vi "daqmx watchdog config UI.vi"() -> ()   [LabVIEW 2014, in "DAQmx Watchdog editor node.lvclass"]
doc: "All child modules share this same UI. The UI allows for the configuration of Channels, Parameters, and Error Handling."
uses:
  DAQmx Watchdog editor node.lvclass
  <vilib>/NI/Configuration Framework/Node/NodeRef.ctl
  <vilib>/NI/Configuration Framework/Node/NISE_CEF_Node.lvclass
  <vilib>/NI/AMC/Message Queue.ctl
  <vilib>/NI/AMC/Message.ctl
  <vilib>/NI/Tools/Keyed Array/KeyedArray.ctl
  <vilib>/NI/Configuration Framework/Node/UserEventRef.ctl
  <vilib>/NI/Configuration Framework/Controls/EventCluster.ctl
  <vilib>/NI/DCAF/Tag Editor Core/control module/configuration/error classification setting.ctl
  <vilib>/NI/Tag Bus Module Framework/runtime/error classification.ctl
  <vilib>/NI/Configuration Framework/Node/RefreshUIEvent.ctl
  <vilib>/NI/Configuration Framework/Node/CacheState.ctl
  <vilib>/NI/Configuration Framework/Node/StopEvent.ctl
  <vilib>/NI/Configuration Framework/Node/NodeChangeEvent.ctl
  <vilib>/NI/DCAF/Tag Editor Core/Table API/Available Tag Menu/channel action event.ctl
  <vilib>/NI/DCAF/Tag Editor Core/Table API/Available Tag Menu/dialog output action.ctl
  <vilib>/NI/Tag Bus Module Framework/channel/TBM channel.lvclass
  <vilib>/NI/Tag Bus/tag/tag descriptor.lvclass
  <vilib>/NI/DCAF/Tag Editor Core/Table API/Table Manager/Call Back Ref Type Def.ctl
  <vilib>/NI/DCAF/Tag Editor Core/Configuration Editor/Classes/Engine Parent/Engine Parent Editor Node.lvclass
  <vilib>/NI/DCAF/Tag Editor Core/Configuration Editor/Classes/Module editor node/module editor node.lvclass
  <vilib>/NI/DCAF/Tag Editor Core/Table API/Table Manager/references.ctl
  <vilib>/NI/DCAF/Tag Editor Core/Table API/Table Manager/Menu Definition.ctl
  <vilib>/NI/DCAF/Tag Editor Core/Table API/Table Manager/Menu Options.ctl
  <vilib>/NI/DCAF/Tag Editor Core/control module/configuration/control module configuration.lvclass
  <vilib>/NI/DCAF/Tag Editor Core/Table API/Table Manager/Table Events.ctl
  <vilib>/NI/DCAF/Tag Editor Core/Table API/Table Manager/Menu Select.ctl
  <vilib>/NI/DCAF/Tag Editor Core/control module/editor node/control module editor.lvclass
  <vilib>/NI/DCAF/Tag Editor Core/control module/configuration/control module configuration.lvclass/control module configuration.ctl
  <vilib>/NI/Configuration Framework/serializable configuration/NISE_CEF_serializable configuration.lvclass/NISE_CEF_serializable configuration.ctl
  <vilib>/NI/Tag Bus Module Framework/channel/channel classification.ctl
  module/configuration/DAQmx Watchdog configuration.lvclass
  <vilib>/NI/DCAF/Tag Editor Core/control module/configuration/Write error classifications.vi
  <vilib>/NI/DCAF/Tag Editor Core/Configuration Editor/Classes/Module editor node/Read Module Configuration.vi
  <vilib>/NI/DCAF/Tag Editor Core/control module/editor node/read fixed channel configuration.vi
  <vilib>/Utility/LVClass/Get LV Class Name.vi
  <vilib>/NI/Configuration Framework/error generator/NISE_error generator.vi
  <vilib>/NI/Tag Bus Module Framework/module configuration/TBM module configuration.lvclass
  <vilib>/NI/Configuration Framework/serializable configuration/NISE_CEF_serializable configuration.lvclass
  <vilib>/NI/DCAF/Tag Editor Core/Table API/Listbox/Multi Column Listbox.lvclass
  <vilib>/NI/Configuration Framework/NISE_CEF_TreeControl.lvlib
  <vilib>/NI/DCAF/Tag Editor Core/Table API/Table Manager.lvlib
  <vilib>/NI/DCAF UI Toolkit/Controls/DCAF UI Elements.lvlib
  <vilib>/NI/Tools/Keyed Array/Tools_KeyedArray.lvlib
  <vilib>/NI/AMC/AMC.lvlib
  <vilib>/NI/DCAF/Tag Editor Core/Table API/Table Manager/Table Manager.lvclass
  <vilib>/NI/Tag Bus Module Framework/runtime/TBM module execution interface.lvclass
panel:
  in  "Enum":i32
  in  "user event out":refnum<user-event>
  in  "Top Level Tab Control":enum32{"Watchdog", "Mapping", "Error Handling"}(tab)
  in  "Trigger on network":bool=TRUE
  in  "Digital States":T1(array[cluster]) caption="Digital Output" {"expiration state" items=["High"=10192, "Low"=10214, "Tristate"=10310, "No Change"=10160]}
  in  "Counter States":T1(array[cluster]) caption="Counter Output" {"expiration state" items=["Low"=10214, "High"=10192, "No Change"=10160]}
  in  "Analog States":T2(array[cluster]) caption="Analog Output" {"output type" items=["Voltage"=10322, "Current"=10134, "No Change"=10160]}
  in  "DAQmx Device Name":tag
  in  "Timeout (s)":dbl=0.01 format="%#_13g"
  in  "Edge":i32(ring)=10280 items=["Rising"=10280, "Falling"=10171]
  in  "Trigger Source":tag
  in  "Trigger Type":i32(ring)=10150 items=["Digital Edge"=10150, "Time"=15996]
  in  "Channels Listbox":i32(listbox)
  in  "mapall":bool
  in  "mapwriters":bool
  in  "error classifications":T3[](array[typedef])
  in  "node change":T5
  in  "stop event":T6
  in  "cache state":T7
  in  "refresh UI":T8
  in  "user event":T9
  in  "main queue":T10
  in  "node ref":T11
  # "Triggering"
  # "Expiration States"
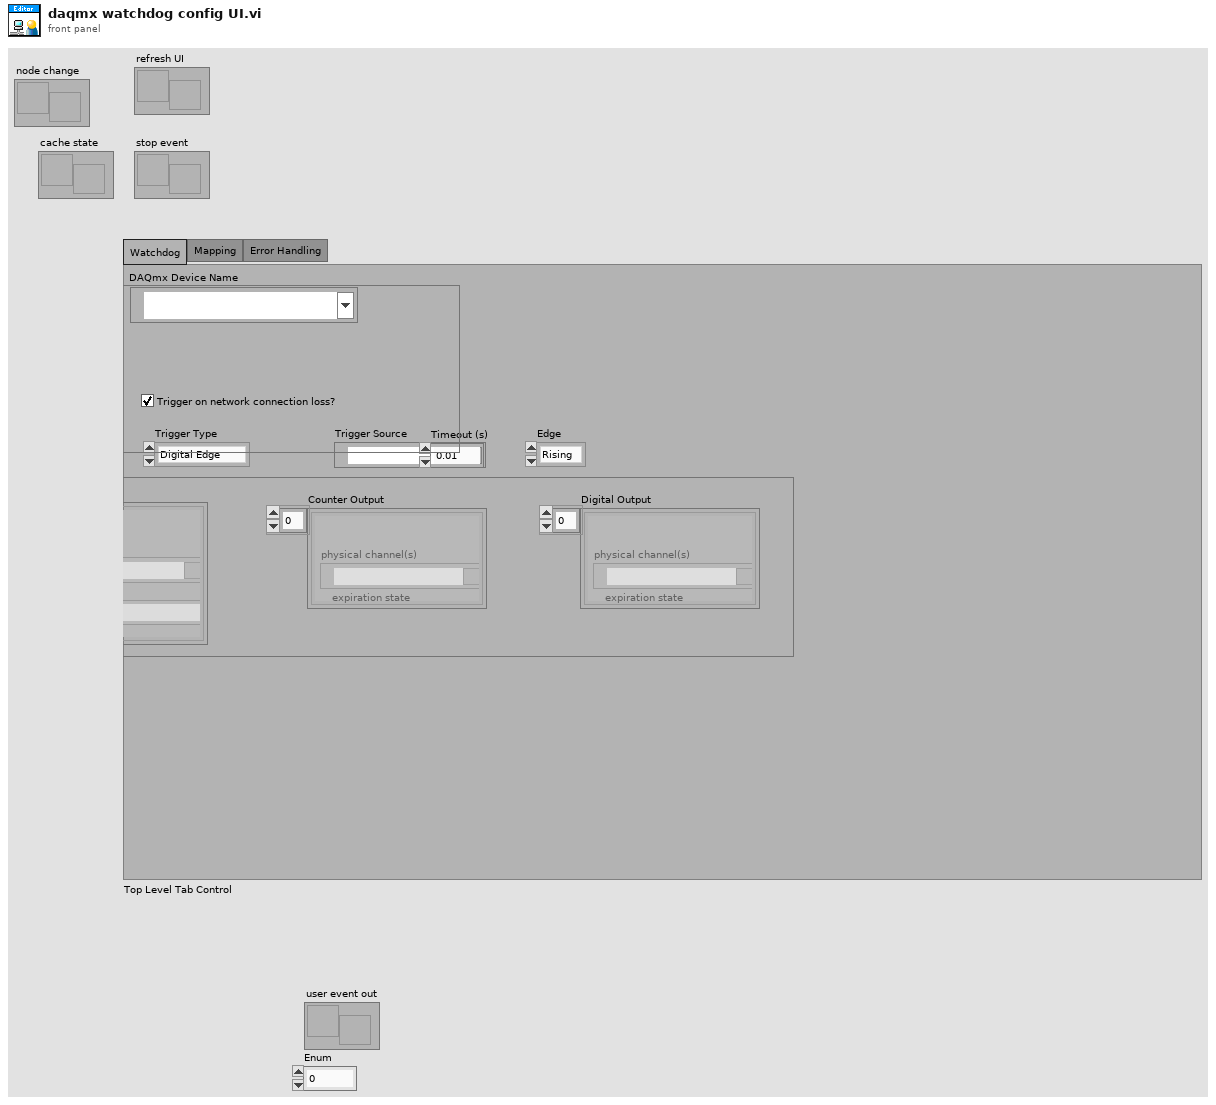
[diagram p1: front panel]
types:
  T1 = cluster{"physical channel(s)":tag, "expiration state":i32}[]
  T2 = cluster{"physical channel":tag, "expiration state":dbl, "output type":i32}[]
  T3 = typedef "control module configuration.lvclass/error classification setting.ctl" = cluster{"code":i32, "error classification":T4}
  T4 = typedef "TBM module execution interface.lvclass/error classification.ctl" = enum16{"unknown", "none", "trivial", "recoverable", "critical"}
  T5 = typedef "NISE_CEF_Node.lvclass/NodeChangeEvent.ctl" = refnum<user-event>
  T6 = typedef "NISE_CEF_Node.lvclass/StopEvent.ctl" = refnum<user-event>
  T7 = typedef "NISE_CEF_Node.lvclass/CacheState.ctl" = refnum<user-event>
  T8 = typedef "NISE_CEF_Node.lvclass/RefreshUIEvent.ctl" = refnum<user-event>
  T9 = typedef "NISE_CEF_Node.lvclass/UserEventRef.ctl" = refnum<user-event>
  T10 = typedef "AMC.lvlib/Message Queue.ctl" = refnum<queue>
  T11 = typedef "NISE_CEF_Node.lvclass/NodeRef.ctl" = refnum<data-value>
  T12 = typedef "Table Manager.lvlib/Table Manager.lvclass/Table Events.ctl" = cluster{"Menu Selection":refnum<user-event>}
  T13 = typedef "Table Manager.lvlib/Table Manager.lvclass/Menu Definition.ctl" = cluster{"Menu Name":string, "Menu Options":T14}
  T14 = typedef "Table Manager.lvlib/Table Manager.lvclass/Menu Options.ctl" = enum16{"Always Show", "Show When Used", "Show When Empty"}
  T15 = typedef "Table Manager.lvlib/Table Manager.lvclass/references.ctl" = cluster{"stop event":T6, "refresh UI":T8, "cache state":T7, "node change":T5, "user event out":refnum<user-event>, "main queue":T10, "user event":T9}
  T16 = typedef "Table Manager.lvlib/Table Manager.lvclass/object ref.ctl" = cluster{"engine":refnum<data-value>, "Node Ref":refnum<data-value>}
  T17 = typedef "Table Manager.lvlib/Column.lvclass/Column Descriptor.ctl" = cluster{"name":string, "caption":string, "Column Type":T18, "Params":string, "AutoSizeMode":i32, "FillWeight":sgl, "MinWidth":u32, "tooltip":string, "Enum Reference":refnum<vi>, "Channel suffix":string, "Read Only":bool, "Call Back VI":T19, "DT Dependency":i32, "name dependency":i32, "data type":T20, "Custom Column":refnum<class "Column.lvclass">}
  T18 = typedef "Table Manager.lvlib/Column.lvclass/Column Type.ctl" = enum16{"String", "Mapping", "Enum", "Custom"}
  T19 = typedef "Table Manager.lvlib/Table Manager.lvclass/Call Back Ref Type Def.ctl" = refnum<vi>
  T20 = typedef "tag bus.lvlib/tag descriptor.lvclass/Data Type.ctl" = enum16{"Double", "Single", "I64", "I32", "I16", "I8", "U64", "U32", "U16", "U8", "Boolean", "String", "Array of Double", "Array of Single", "Array of I64", "Array of I32", "Array of I16", "Array of I8", "Array of U64", "Array of U32", "Array of U16", "Array of U8", "Array of Boolean", "Array of String"}
  T21 = typedef "NISE_CEF_TreeControl.lvlib/EventCluster.ctl" = cluster{"command":string, "data":string}
  T22 = typedef "TBM channel.lvclass/channel classification.ctl" = enum16{"input data", "output data", "processing parameter", "processing result"}
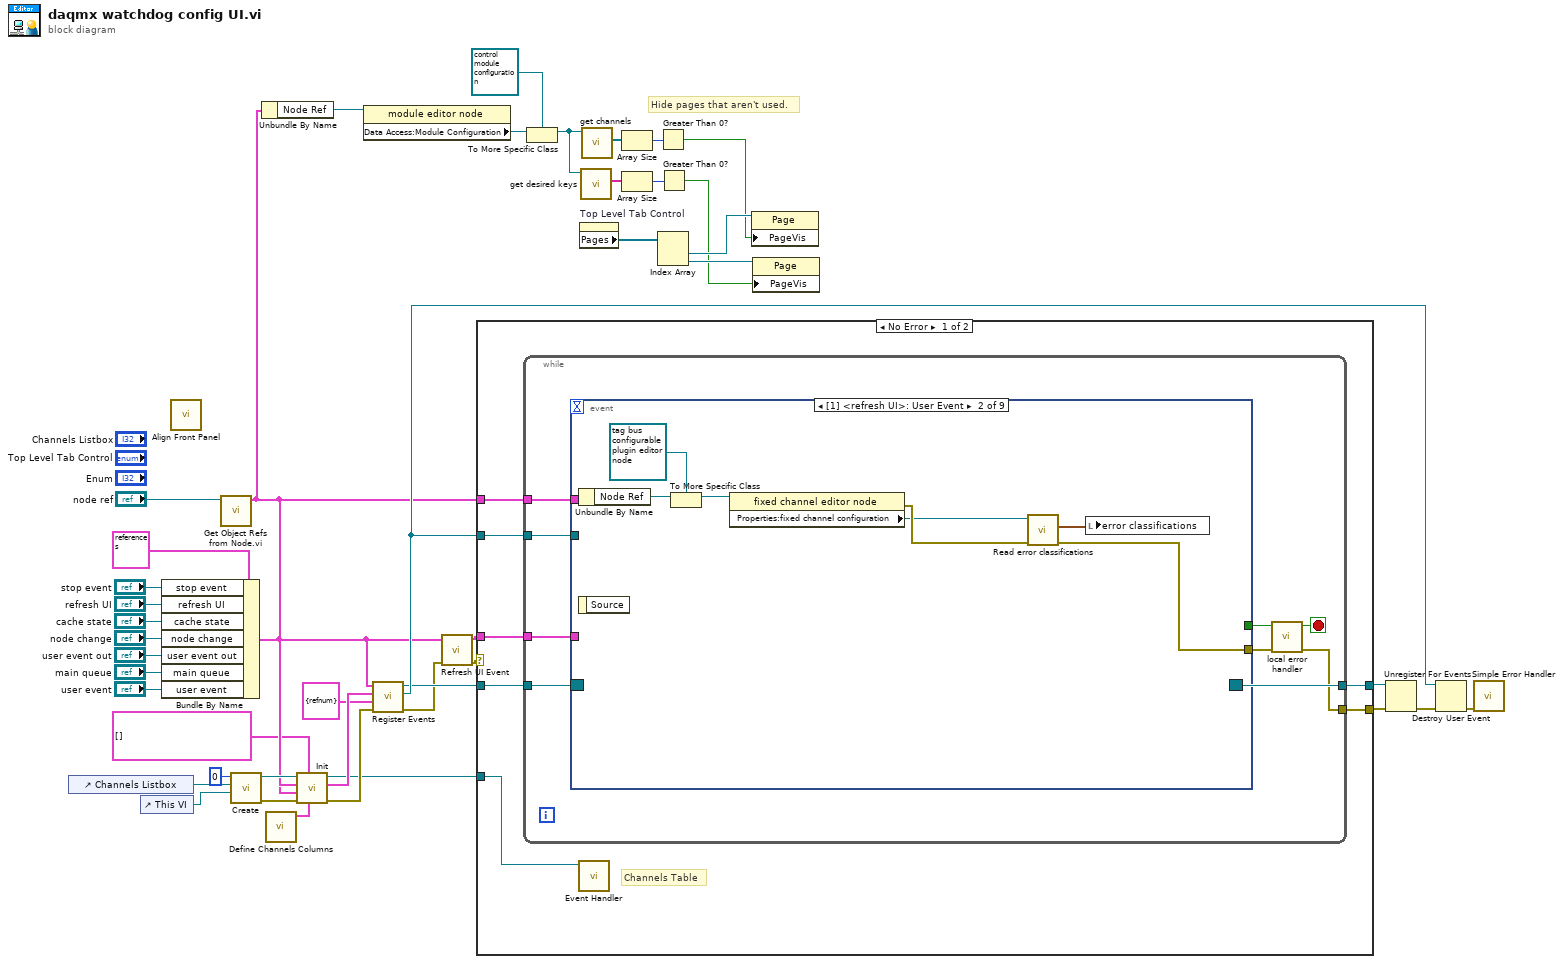
[diagram p0: block diagram]
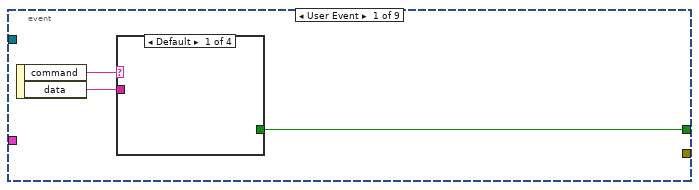
[diagram p2: hidden frame]
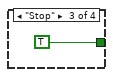
[diagram p4: hidden frame]
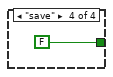
[diagram p5: hidden frame]
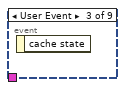
[diagram p6: hidden frame]
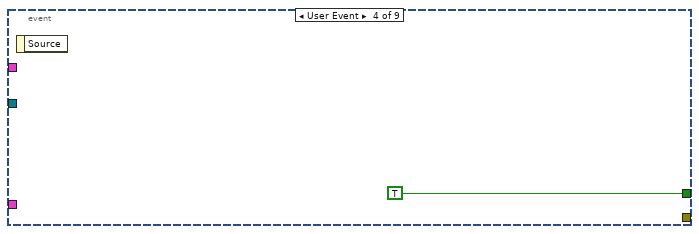
[diagram p7: hidden frame]
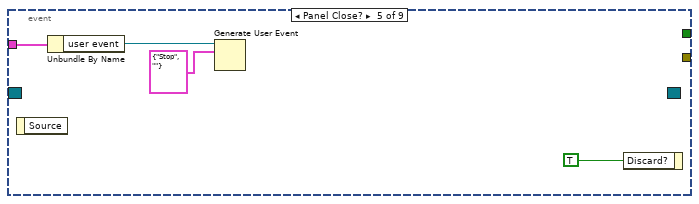
[diagram p8: hidden frame]
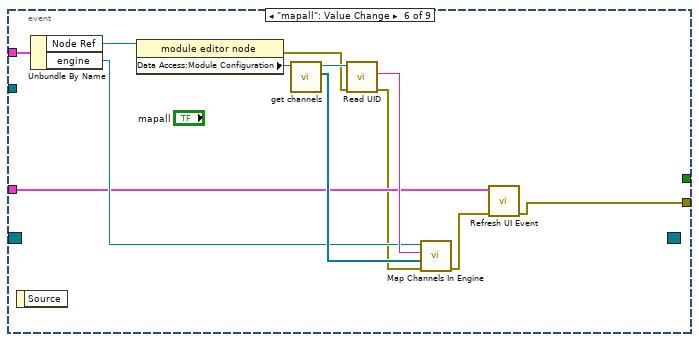
[diagram p9: hidden frame]
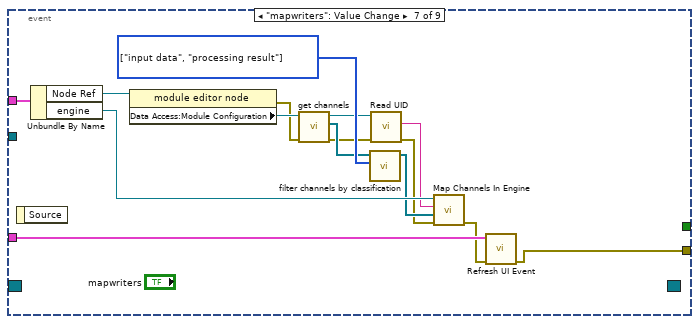
[diagram p10: hidden frame]
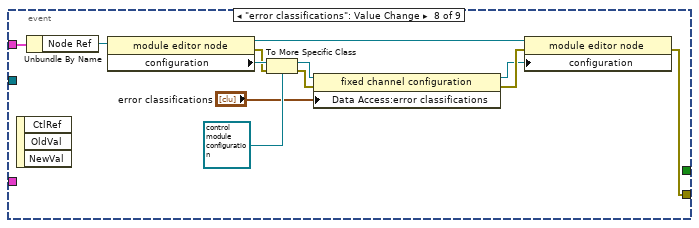
[diagram p11: hidden frame]
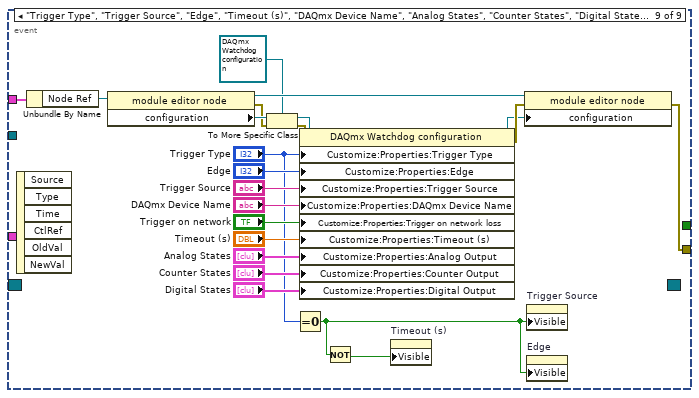
[diagram p12: hidden frame]
diagram:
  # "Hide pages that aren't used."
  n1 = control-ref of="Channels Listbox"() -> (w20:refnum<vi>)
  n2 = control-ref of="This VI"() -> (w19:refnum<vi>)
  n3 = Bundle By Name(cluster=T15 {"stop event"=refnum, "refresh UI"=refnum, "cache state"=refnum, "node change"=refnum, "user event out"=refnum, "main queue"=refnum, "user event"=refnum} ("Event References"), "stop event"="stop event", "refresh UI"="refresh UI", "cache state"="cache state", "node change"="node change", "user event out"="user event out", "main queue"="main queue", "user event"="user event") -> (w18:T15)
  n4 = call <vilib>:"Align Front Panel.vi"() -> ()  [unwired: 10 in, 2 out]
  n5 = call <vilib>:"Get Object Refs from Node.vi.vi"("node ref"="node ref") -> ("Node object refs"=w8:T16)  [unwired: 9 in, 1 out]
  n6 = call <vilib>:"Create.vi"("Top VI"=w19, "Listbox"=w20, "Index"=0) -> ("error out"=w23:errorcluster, "reference out"=w24:refnum<class "Multi Column Listbox.lvclass">)  [unwired: 7 in]
  n7 = Unbundle By Name(w8) -> ("Node Ref"=w6:refnum<data-value>)
  n8 = call <vilib>:"Define Channels Columns.vi"() -> ("Column Descriptors"=w17:T17[])  [unwired: 11 in]
  n9 = call-dynamic "Init.vi"("Column Descriptors"=w17, "Right-Click Menu"=T13[] [], "error in (no error)"=w23, "Node object refs"=w8, "Event References"=w18, "Multi Column Listbox in"=w24) -> ("error out"=w22:errorcluster, "Table Events"=w34:T12, "Multi Column Listbox out"=w21:refnum<class "Multi Column Listbox.lvclass">)  [unwired: 3 in]
  n10 = property class="module editor node"(reference=w6) -> ("Data Access:Module Configuration"=w7:refnum<class "TBM module configuration.lvclass">)  [unwired: 1 in, 2 out]
  n11 = call <vilib>:"Register Events.vi"("error in (no error)"=w22, "Parameters Table Events"=T12 {"Menu Selection"=refnum}, "Channels Table Events"=w34, "Event References"=w18) -> ("error out"=w27:errorcluster, "Channel Action"=w33:refnum<user-event>, "Event Registration Refnum"=w32:refnum<event-registration>)  [unwired: 5 in]
  n12 = call <vilib>:"Refresh UI Event.vi"("error in (no error)"=w27, "Event References"=w18) -> ("error out"=w28:errorcluster, "Event References out"=w26:T15)  [unwired: 8 in]
  n13 = case shown="No Error" w28 {
    selector: w28 -> [_ w140]
    tunnel: w32 -> [w51 w139]
    tunnel: [w50 w139] -> w44
    tunnel: [w48 w140] -> w43
    tunnel: w33 -> [w49 _]
    tunnel: w8 -> [w47 _]
    tunnel: w26 -> [w46 _]
    tunnel: w21 -> [w45 _]
    frame No Error {
      # "Channels Table"
      n14 = while {
        tunnel: w51 -> [w60]
        tunnel: [w59] -> w50
        tunnel: w49 -> [w58]
        tunnel: [w54] -> w48
        tunnel: w47 -> [w53]
        tunnel: w46 -> [w52]
        stop <- w56 stop-if-true
        n15 = event shown="[1] <refresh UI>: User Event" {
          selector: w60 -> [_ _ _ _ _ _ _ _ _]
          dyn-events: [_ _ _ _ _ _ _ _ _] -> w59
          timeout: _ -> [_ _ _ _ _ _ _ _ _]
          tunnel: [w63 _ _ TRUE _ _ _ _ _] -> w57
          tunnel: [_ w70 _ _ _ w84 w100 w116 w138] -> w55
          tunnel: w58 -> [_ _ _ _ _ _ _ _ _]
          tunnel: w53 -> [_ w73 _ _ _ w88 w101 w115 w137]
          tunnel: w52 -> [_ _ _ _ w76 w83 w99 _ _]
          event User Event {
            n16 = event-data() -> ("command"=w62:string, "data"=w61:string)  [unwired: 1 in]
            n17 = case shown="Default" w62 {
              tunnel: [_ _ TRUE FALSE] -> w63
              tunnel: w61 -> [_ _ _ _]
              frame Default {
              }
              frame "Refresh" {
              }
              frame "Stop" {
              }
              frame "save" {
              }
            }
          }
          event User Event {
            n18 = Unbundle By Name(w73) -> ("Node Ref"=w71:refnum<data-value>)
            n19 = event-data() -> ()  [unwired: 1 in, 1 out]
            n20 = To More Specific Class(target class=refnum<data-value> refnum ("data value reference"), reference=w71) -> (specific class reference=w69:refnum<data-value>)  [unwired: 1 in, 1 out]
            n21 = property class="fixed channel editor node"(reference=w69) -> (error out=w68:errorcluster, "Properties:fixed channel configuration"=w66:refnum<class "control module configuration.lvclass">)  [unwired: 1 in, 1 out]
            n22 = call <vilib>:"Read error classifications.vi"("error in"=w68, "control module configuration in"=w66) -> ("error out"=w70:errorcluster, "error classifications"=w67:T3[])  [unwired: 7 in, 1 out]
            n23 = local write "error classifications"(w67) -> ()
          }
          event User Event {
            n24 = event-data() -> ()  [unwired: 1 in, 1 out]
          }
          event User Event {
            n25 = event-data() -> ()  [unwired: 1 in, 1 out]
          }
          event Panel Close? {
            n26 = event-data() -> ()  [unwired: 1 in, 1 out]
            n27 = Unbundle By Name(w76) -> ("user event"=w75:T9)
            n28 = Generate User Event(user event=w75, event data cluster=T21 {"command"="Stop", "data"=""} ("event data")) -> ()  [unwired: 2 in, 2 out]
            n29 = event-data("Discard?"=TRUE) -> ()  [unwired: 1 in, 1 out]
          }
          event "mapall": Value Change {
            n30 = event-data() -> ()  [unwired: 1 in, 1 out]
            n31 = Unbundle By Name(w88) -> ("Node Ref"=w87:refnum<data-value>, "engine"=w86:refnum<data-value>)
            n32 = property class="module editor node"(reference=w87) -> (error out=w80:errorcluster, "Data Access:Module Configuration"=w82:refnum<class "TBM module configuration.lvclass">)  [unwired: 1 in, 1 out]
            n33 = call-dynamic "get channels.vi"("module configuration in"=w82) -> ("channels"=w90:refnum<class "TBM channel.lvclass">[], "module configuration out"=w81:refnum<class "TBM module configuration.lvclass">)  [unwired: 9 in]
            n34 = call <vilib>:"Read UID.vi"("error in"=w80, "configuration in"=w81) -> ("error out"=w79:errorcluster, "instance id"=w89:string)  [unwired: 7 in, 1 out]
            n35 = call <vilib>:"Map Channels In Engine.vi"("error in (no error)"=w79, "channels"=w90, "instance id"=w89, "Engine DVR"=w86) -> ("error out"=w85:errorcluster)  [unwired: 7 in]
            n36 = call <vilib>:"Refresh UI Event.vi"("error in (no error)"=w85, "Event References"=w83) -> ("error out"=w84:errorcluster)  [unwired: 8 in, 1 out]
          }
          event "mapwriters": Value Change {
            w104 = T22[] [enum."input data", enum."processing result"] items=["input data", "output data", "processing parameter", "processing result"] ("allowed classifications")
            n37 = event-data() -> ()  [unwired: 1 in, 1 out]
            n38 = Unbundle By Name(w101) -> ("Node Ref"=w102:refnum<data-value>, "engine"=w98:refnum<data-value>)
            n39 = property class="module editor node"(reference=w102) -> (error out=w91:errorcluster, "Data Access:Module Configuration"=w93:refnum<class "TBM module configuration.lvclass">)  [unwired: 1 in, 1 out]
            n40 = call-dynamic "get channels.vi"("module configuration in"=w93) -> ("channels"=w103:refnum<class "TBM channel.lvclass">[], "module configuration out"=w92:refnum<class "TBM module configuration.lvclass">)  [unwired: 9 in]
            n41 = call <vilib>:"filter channels by classification.vi"("allowed classifications"=w104, "channels in"=w103) -> ("channels out"=w96:refnum<class "TBM channel.lvclass">[])  [unwired: 9 in]
            n42 = call <vilib>:"Read UID.vi"("error in"=w91, "configuration in"=w92) -> ("error out"=w95:errorcluster, "instance id"=w97:string)  [unwired: 7 in, 1 out]
            n43 = call <vilib>:"Map Channels In Engine.vi"("error in (no error)"=w95, "channels"=w96, "instance id"=w97, "Engine DVR"=w98) -> ("error out"=w94:errorcluster)  [unwired: 7 in]
            n44 = call <vilib>:"Refresh UI Event.vi"("error in (no error)"=w94, "Event References"=w99) -> ("error out"=w100:errorcluster)  [unwired: 8 in, 1 out]
          }
          event "error classifications": Value Change {
            n45 = event-data() -> ()  [unwired: 1 in, 3 out]
            n46 = Unbundle By Name(w115) -> ("Node Ref"=w110:refnum<data-value>)
            n47 = property class="module editor node"(reference=w110) -> (reference out=w114:refnum<data-value>, error out=w106:errorcluster, "configuration"=w109:refnum<class "NISE_CEF_serializable configuration.lvclass">)  [unwired: 1 in]
            n48 = To More Specific Class(target class=refnum<class "control module configuration.lvclass"> refnum ("fixed channel configuration"), reference=w109, error in=w106) -> (specific class reference=w111:refnum<class "control module configuration.lvclass">, error out=w105:errorcluster)
            n49 = property class="fixed channel configuration"(reference=w111, error in=w105, "Data Access:error classifications"="error classifications") -> (reference out=w112:refnum<class "control module configuration.lvclass">, error out=w113:errorcluster)
            n50 = property class="module editor node"(reference=w114, error in=w113, "configuration"=w112) -> (error out=w116:errorcluster)  [unwired: 1 out]
          }
          event "Trigger Type", "Trigger Source", "Edge", "Timeout (s)", "DAQmx Device Name", "Analog States", "Counter States", "Digital States", "Trigger on network": Value Change {
            n51 = event-data() -> ()  [unwired: 1 in, 6 out]
            n52 = Unbundle By Name(w137) -> ("Node Ref"=w132:refnum<data-value>)
            n53 = property class="module editor node"(reference=w132) -> (reference out=w136:refnum<data-value>, error out=w129:errorcluster, "configuration"=w131:refnum<class "NISE_CEF_serializable configuration.lvclass">)  [unwired: 1 in]
            n54 = To More Specific Class(target class=refnum<class "DAQmx Watchdog configuration.lvclass"> refnum ("DAQmx Watchdog configuration"), reference=w131, error in=w129) -> (specific class reference=w133:refnum<class "DAQmx Watchdog configuration.lvclass">, error out=w128:errorcluster)
            n55 = Equal To 0?(x="Trigger Type") -> (x = 0?=w117:bool)
            n56 = property class="DAQmx Watchdog configuration"(reference=w133, error in=w128, "Customize:Properties:Trigger Type"="Trigger Type", "Customize:Properties:Edge"="Edge", "Customize:Properties:Trigger Source"="Trigger Source", "Customize:Properties:DAQmx Device Name"="DAQmx Device Name", "Customize:Properties:Trigger on network loss"="Trigger on network", "Customize:Properties:Timeout (s)"="Timeout (s)", "Customize:Properties:Analog Output"="Analog States", "Customize:Properties:Counter Output"="Counter States", "Customize:Properties:Digital Output"="Digital States") -> (reference out=w134:refnum<class "DAQmx Watchdog configuration.lvclass">, error out=w135:errorcluster)
            n57 = Not(x=w117) -> (.not. x?=w118:bool)
            n58 = property on="Timeout (s)" class="DigNum (strict)"("Visible"=w118) -> ()  [unwired: 2 in, 2 out]
            n59 = property class="module editor node"(reference=w136, error in=w135, "configuration"=w134) -> (error out=w138:errorcluster)  [unwired: 1 out]
            n60 = property on="Trigger Source" class="DAQmxName"("Visible"=w117) -> ()  [unwired: 2 in, 2 out]
            n61 = property on="Edge" class="Ring (strict)"("Visible"=w117) -> ()  [unwired: 2 in, 2 out]
          }
        }
        n62 = call <vilib>:"local error handler.vi"("error in (no error)"=w55, "Stop in"=w57) -> ("error out"=w54:errorcluster, "Stop out"=w56:bool)  [unwired: 8 in]
      }
      n63 = call-dynamic "Event Handler.vi"("Listbox in"=w45) -> ()  [unwired: 9 in, 2 out]
    }
    frame Error {
    }
  }
  n64 = To More Specific Class(target class=refnum<class "control module configuration.lvclass"> refnum ("fixed channel configuration"), reference=w7) -> (specific class reference=w4:refnum<class "control module configuration.lvclass">)  [unwired: 1 in, 1 out]
  n65 = property on="Top Level Tab Control" class="TabCtl (strict)"() -> ("Pages"=w9:refnum<vi>[])  [unwired: 2 in, 2 out]
  n66 = call-dynamic "get desired keys.vi"("fixed channel configuration in"=w4) -> ("desired keys"=w12:string[])  [unwired: 8 in, 2 out]
  n67 = call-dynamic "get channels.vi"("fixed channel configuration in"=w4) -> ("channels"=w15:refnum<class "TBM channel.lvclass">[])  [unwired: 9 in, 1 out]
  n68 = Array Size(array=w15) -> (size(s)=w14:i32)
  n69 = Array Size(array=w12) -> (size(s)=w13:i32)
  n70 = Greater Than 0?(x=w14) -> (x > 0?=w3:bool)
  n71 = Index Array(array=w9) -> (element #1=w10:refnum<vi>, element #2=w11:refnum<vi>)  [unwired: 2 in]
  n72 = Greater Than 0?(x=w13) -> (x > 0?=w2:bool)
  n73 = property class="Page"(reference=w10, "PageVis"=w3) -> ()  [unwired: 1 in, 2 out]
  n74 = property class="Page"(reference=w11, "PageVis"=w2) -> ()  [unwired: 1 in, 2 out]
  n75 = Unregister For Events(event registration refnum=w44, error in=w43) -> (error out=w42:errorcluster)
  n76 = Destroy User Event(user event=w33, error in=w42) -> (error out=w41:errorcluster)
  n77 = call <vilib>:"Simple Error Handler.vi"("error in (no error)"=w41) -> ()  [unwired: 4 in, 5 out]
